vi "Calib_Ch_setup.vi"(4 "Ch & spans":T2[](array[typedef])=[{"Ch No"=1, "Var name"="Cross wire 1", "Device"="", "Port"=""}, {"Ch No"=2, "Var name"="Cross wire 2", "Device"="", "Port"=""}] {"Ch No" min=0 max=7}, 6 "Calib filename":path) -> (0 "Output string":string)   [LabVIEW 2022 SP3]
uses:
  Calib Channel Setup.ctl
  Controls/Inst_type.ctl
  Controls/Analysis_info_cluster.ctl
  Controls/Instrument_Array.ctl
  Controls/channelState.ctl
  Globals/Meas_global.vi
panel:
  in  "Inst type":T1
  out "length":i32
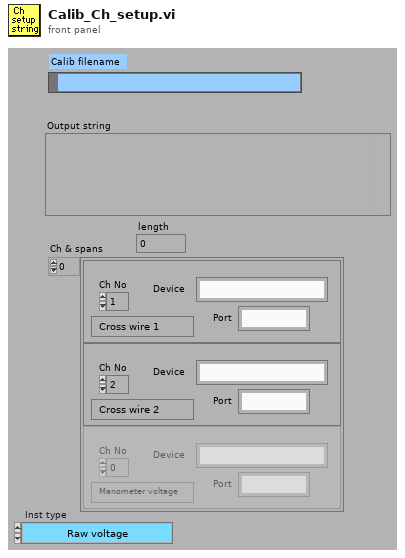
[diagram p1: front panel]
types:
  T1 = typedef "Inst_type.ctl" = enum16{"Raw voltage", "Raw with zero offsetting", "Propeller anemometer", "Pressure Transducer", "Pitot-static tube", "Hot wire", "Cross wire 1", "Cross wire 2", "Generic Linear", "Generic Polynomial", "Generic BackPoly", "Fast FID", "Thermocouple", "Cold wire", "Pulsed Wire", "LDA Vel", "LDA Tran time", "LDA Arr time", "Microphone"}
  T2 = typedef "Calib Channel Setup.ctl" = cluster{"Ch No":i16, "Var name":string, "Device":string, "Port":string}
  T3 = typedef "Analysis_info_cluster.ctl" = cluster{"Colour":u32, "Inst type":T1, "Inst name":string, "Symbol":string, "Code name":string, "Extra Info":string, "Inst Array":T4, "U":dbl, "u^2":dbl, "u^3":dbl, "u^4":dbl, "Skew_u":dbl, "Kurt_u":dbl, "Sd Error in Mean":dbl, "% u'/U":dbl, "X":dbl, "Y":dbl, "Z":dbl, "Timescale integral Estimate":dbl, "Sd Error in Variance":dbl, "Calib File":path, "Calib Constants":dbl[], "Output Position":bool, "Stats":enum16{"None", "Basic", "Full"}, "Av Sampling Rate":dbl, "Av No of Samples":dbl, "Total Meas Time (s)":dbl, "OrigChName":string, "Max value":dbl, "Min value":dbl, "Req Sample Rate Hz":dbl, "Sync Delay Time (s)":dbl, "Ch No":i16, "Device":string, "Use Latest Calib":bool, "Port":string, "Metadata Ch Names":string[], "Metadata Ch Values":string[], "Label":string, "chState":T5, "Point Drift":dbl, "inputConfig":string}
  T4 = typedef "Instrument_Array.ctl" = enum16{"PWA", "LDA", "Analogue"}
  T5 = typedef "channelState.ctl" = enum32{"No Selection", "Solo", "Mute"}
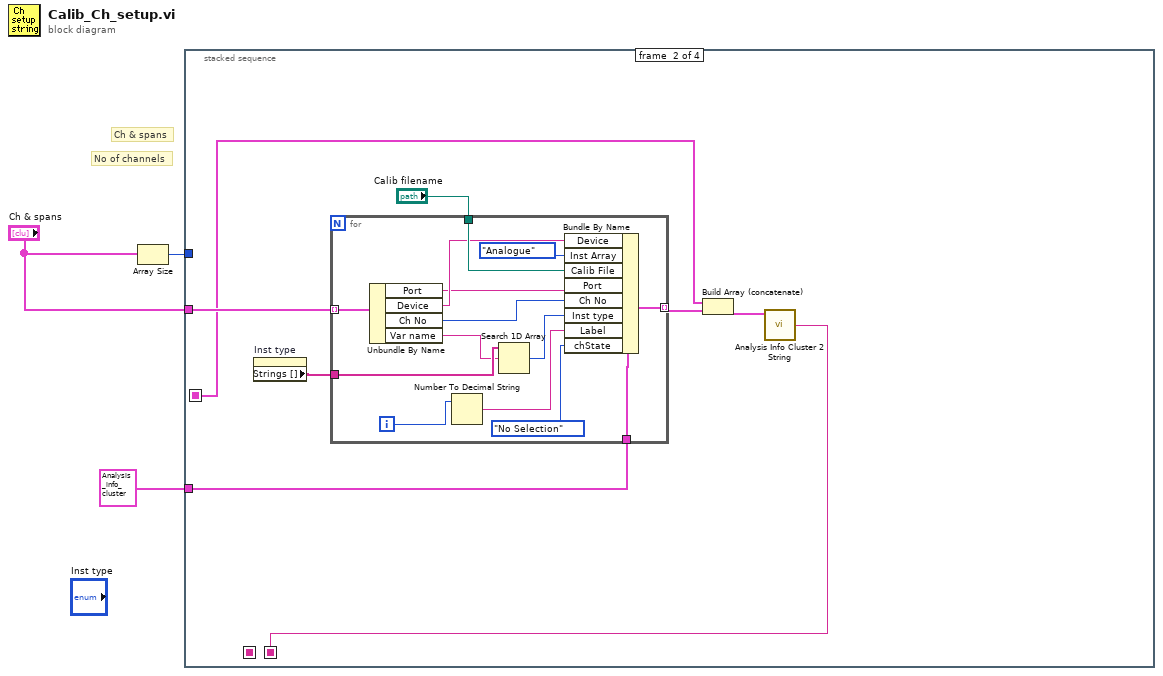
[diagram p0: block diagram]
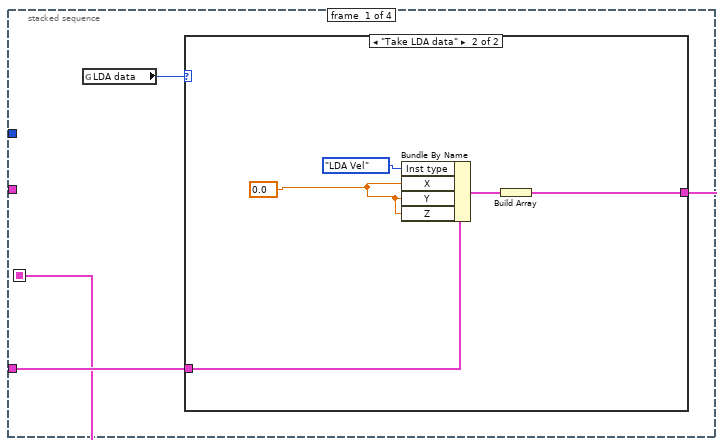
[diagram p2: hidden frame]
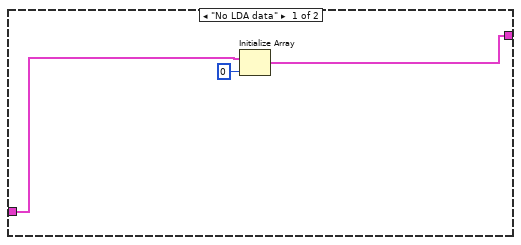
[diagram p3: hidden frame]
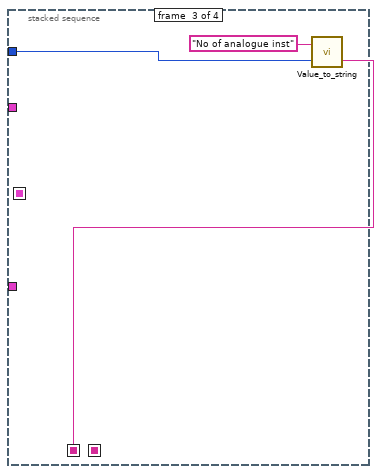
[diagram p4: hidden frame]
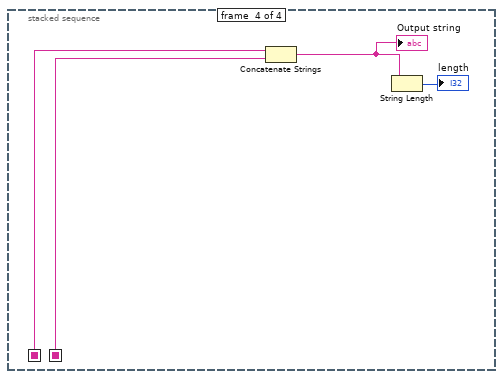
[diagram p5: hidden frame]
diagram:
  # "No of channels"
  # "Ch & spans"
  n1 = Array Size(array="Ch & spans") -> (size(s)=w2:i32)
  n2 = stacked-sequence {
    seq-local: [_ w20 _ _] -> [_ _ _ w40]
    seq-local: [_ _ w37 _] -> [_ _ _ w41]
    seq-local: [w4 _ _ _] -> [_ w17 _ _]
    tunnel: "Ch & spans" -> [_ w19 _ _]
    tunnel: w2 -> [_ _ w38 _]
    tunnel: T3 {"Colour"=0, "Inst type"=enum."Pitot-static tube", "Inst name"="Manometer voltage", "Symbol"="U", "Code name"="", "Extra Info"="U", "Inst Array"=enum."PWA", "U"=0.0, "u^2"=0.0, "u^3"=0.0, "u^4"=0.0, "Skew_u"=0.0, "Kurt_u"=0.0, "Sd Error in Mean"=0.0, "% u'/U"=0.0, "X"=0.0, "Y"=0.0, "Z"=0.0, "Timescale integral Estimate"=0.0, "Sd Error in Variance"=0.0, "Calib File"=path "", "Calib Constants"=[], "Output Position"=FALSE, "Stats"=enum."None", "Av Sampling Rate"=0.0, "Av No of Samples"=0.0, "Total Meas Time (s)"=0.0, "OrigChName"="", "Max value"=0.0, "Min value"=0.0, "Req Sample Rate Hz"=0.0, "Sync Delay Time (s)"=0.0, "Ch No"=0, "Device"="", "Use Latest Calib"=FALSE, "Port"="", "Metadata Ch Names"=[], "Metadata Ch Values"=[], "Label"="", "chState"=enum."Solo", "Point Drift"=0.0, "inputConfig"=""} -> [w5 w18 _ _]
    frame #0 {
      n3 = global read "Meas_global.vi" "LDA data"() -> (w6:enum16{"No LDA data", "Take LDA data"})
      n4 = case shown="\"Take LDA data\"" w6 {
        tunnel: w5 -> [w8 w11]
        tunnel: [w7 w10] -> w4
        frame "No LDA data" {
          n5 = Initialize Array(w8, 0 ("dimension size")) -> (w7:T3[])
        }
        frame "Take LDA data" {
          w13 = 0.0 ("X")
          n6 = Bundle By Name(cluster=w11, "Inst type"=Inst_type."LDA Vel", "X"=w13, "Y"=w13, "Z"=w13) -> (w14:T3)
          n7 = Build Array(w14) -> (w10:T3[])
        }
      }
    }
    frame #1 {
      n8 = property on="Inst type" class="Enum (strict)"() -> ("Strings []"=w22:string[])  [unwired: 2 in, 2 out]
      n9 = for {
        tunnel: w19 -> [w36] mode=indexing
        tunnel: w22 -> [w34]
        tunnel: [w31] -> w16 mode=indexing
        tunnel: "Calib filename" -> [w28]
        tunnel: w18 -> [w26]
        i -> [w30]
        n10 = Unbundle By Name(w36) -> ("Port"=w24:string, "Device"=w25:string, "Ch No"=w35:i16, "Var name"=w33:string)
        n11 = Number To Decimal String(number=w30) -> (decimal integer string=w29:string)  [unwired: 1 in]
        n12 = Search 1D Array(1D array=w34, element=w33) -> (index of element=w32:i32)  [unwired: 1 out]
        n13 = Bundle By Name(cluster=w26, "Device"=w25, "Inst Array"=Instrument_Array."Analogue", "Calib File"=w28, "Port"=w24, "Ch No"=w35, "Inst type"=w32, "Label"=w29, "chState"=channelState."No Selection") -> (w31:T3)
      }
      n14 = Build Array (concatenate)(w17, w16) -> (w15:T3[])
      n15 = call "Analysis Info Cluster 2 String.vi"("Analysis Info cluster"=w15) -> ("Output string"=w20:string)  [unwired: 5 in]
    }
    frame #2 {
      n16 = call "Value_to_string.vi"("Value"=w38, "Label for value"="No of analogue inst") -> ("Output string"=w37:string)  [unwired: 1 in]
    }
    frame #3 {
      n17 = Concatenate Strings(w41, w40) -> (w42:string)
      "Output string" <- w42
      n18 = String Length(string=w42) -> (length=→"length":i32)
    }
  }
